vi "Initialize.vi"(8 "error in (no error)":errorcluster, 11 "Config in":refnum<class "JSON Variable.lvclass">) -> (0 "error out":errorcluster, 3 "Config out":refnum<class "JSON Variable.lvclass">)   [LabVIEW 2019, in "JSON Variable.lvclass"]
uses:
  JSON Variable.lvclass
  JSON Variable.lvclass/JSON Variable.ctl
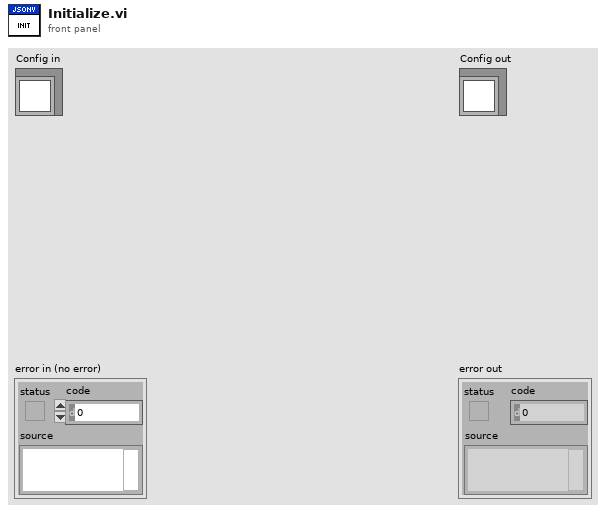
[diagram p1: front panel]
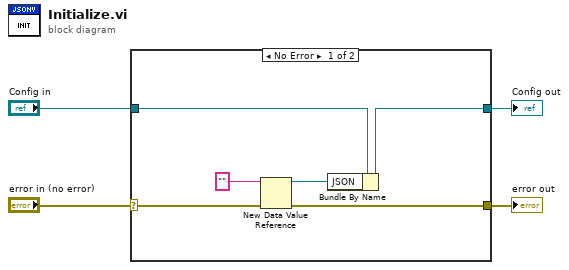
[diagram p0: block diagram]
diagram:
  n1 = case shown="No Error" "error in (no error)" {
    selector: "error in (no error)" -> [w6 w12]
    tunnel: [w5 w12] -> w3
    tunnel: [w8 w11] -> w1
    tunnel: "Config in" -> [w10 w11]
    frame No Error {
      n2 = New Data Value Reference(data value="", error in=w6) -> (data value reference=w7:refnum<data-value>, error out=w5:errorcluster)
      n3 = Bundle By Name(cluster=w10, "JSON"=w7) -> (w8:refnum<class "JSON Variable.lvclass">)
    }
    frame Error {
    }
  }
  "error out" <- w3
  "Config out" <- w1
